vi "Start Sequence Acquisition.vi"(8 "error in (no error)":errorcluster, 11 "DAQ in":refnum<class "DAQ.lvclass">) -> (0 "error out":errorcluster, 3 "DAQ out":refnum<class "DAQ.lvclass">)   [LabVIEW 2020, in "DAQ.lvlib" / "DAQ.lvclass"]
uses:
  DAQ.lvclass
  C:/Program Files/National Instruments/LabVIEW 2020/vi.lib/ActorFramework/Actor/Actor.lvclass
  DAQ.lvclass/DAQ.ctl
  <vilib>/ActorFramework/Actor/Actor.lvclass/Actor.ctl
  <vilib>/ActorFramework/Message Enqueuer/Message Enqueuer.lvclass/Message Enqueuer.ctl
  <vilib>/ActorFramework/Message Enqueuer/Init from Existing Queue.vi
  <vilib>/ActorFramework/Message Enqueuer/Enqueue.vi
  DAQ Messages/Start Sequence Acquisition Msg/Start Sequence Acquisition Msg.lvclass
  C:/Program Files/National Instruments/LabVIEW 2020/vi.lib/ActorFramework/Message/Message.lvclass
  <vilib>/ActorFramework/Message Priority Queue/Priority Enqueue.vi
  <vilib>/ActorFramework/Message Enqueuer/Message Enqueuer.lvclass
  <vilib>/ActorFramework/Actor/Actor.lvclass
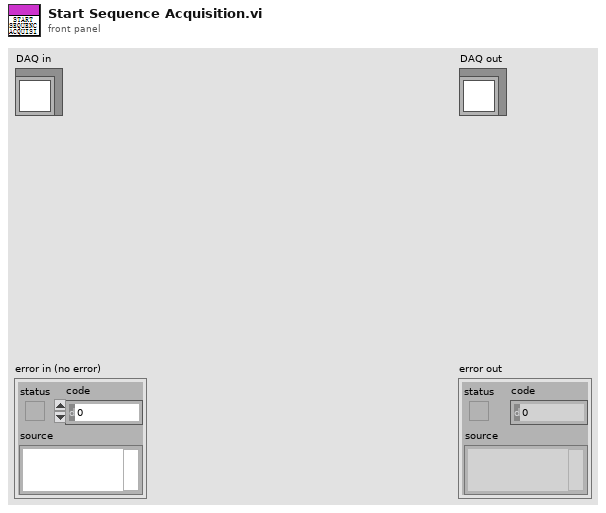
[diagram p1: front panel]
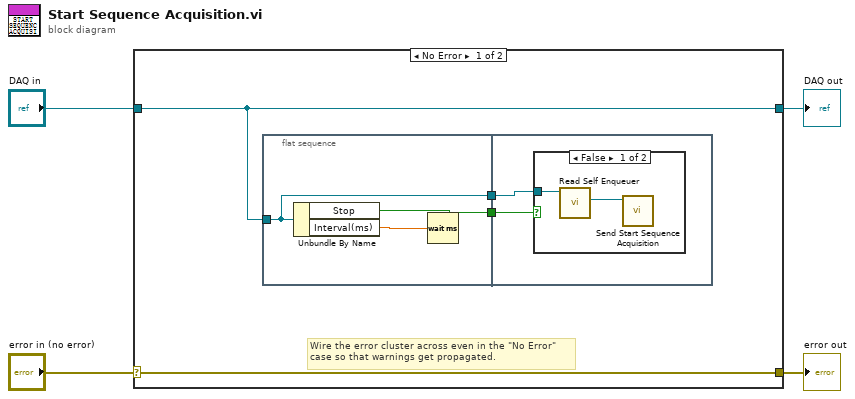
[diagram p0: block diagram]
diagram:
  n1 = case shown="No Error" "error in (no error)" {
    selector: "error in (no error)" -> [w8 w17]
    tunnel: [w8 w17] -> w3
    tunnel: [w7 w16] -> w1
    tunnel: "DAQ in" -> [w7 w16]
    frame No Error {
      # "Wire the error cluster across even in the \"No Error\"\ncase so that warnings get propagated."
      n2 = flat-sequence {
        tunnel: w7 -> [w9]
        tunnel: [w10] -> w6
        tunnel: [w9] -> w5
        tunnel: w6 -> [w12]
        tunnel: w5 -> [w13]
        frame #0 {
          n3 = Unbundle By Name(w9) -> ("Stop"=w10:bool, "Interval(ms)"=w11:dbl)
          n4 = Wait (ms)(milliseconds to wait=w11) -> ()  [unwired: 1 out]
        }
        frame #1 {
          n5 = case shown="False" w12 {
            tunnel: w13 -> [w15 _]
            frame False {
              n6 = call <vilib>:"Read Self Enqueuer.vi"("Actor"=w15) -> ("Self Enqueuer"=w14:refnum<class "Message Enqueuer.lvclass">)  [unwired: 10 in]
              n7 = call "Send Start Sequence Acquisition.vi"("Message Enqueuer"=w14) -> ()  [unwired: 9 in, 2 out]
            }
            frame True {
            }
          }
        }
      }
    }
    frame Error {
    }
  }
  "error out" <- w3
  "DAQ out" <- w1
